vi "Start Stream.vi"(8 "error in (no error)":errorcluster, 10 "Camera Settings":T1={"Exposure Time (ms)"=100.0, "Binning"=enum."2x2", "Scan Mode"=0, "Frames to Acquire"=1000.0, "Pixel Correction"=FALSE, "Frames to Skip"=0, "File Path"=path "", "Duty cycle"=0.0, "ALEX"=FALSE, "Shutter Enable"=[], "fluidics trigger frame"=0, "Bit Depth"=16, "Image Width (px)"=0, "Image Height (px)"=0, "Horizontal Offset (px)"=0, "Vertical Offset (px)"=0} {"fluidics trigger frame" max=60000 step=1; "Exposure Time (ms)" min=1.0 max=10000.0 step=1.0}, 11 "Camera in":refnum<class "Camera.lvclass">) -> (0 "error out":errorcluster, 3 "Camera out":refnum<class "Camera.lvclass">)   [LabVIEW 2023, in "Camera.lvlib" / "Camera.lvclass"]
uses:
  Camera.lvclass
  Resources/Type Defs/Camera Settings.ctl
  Camera.lvclass/Camera.ctl
  <vilib>/Utility/error.llb/DialogType.ctl
  <vilib>/ActorFramework/Actor/Actor.lvclass/Actor.ctl
  <vilib>/ActorFramework/Message Enqueuer/Message Enqueuer.lvclass/Message Enqueuer.ctl
  <vilib>/ActorFramework/Message Enqueuer/Enqueue.vi
  Application Messages/Record Button Off Msg/Cancel Operation Msg.lvclass
  Resources/GLOBAL/GLOBAL Time-critical.vi
  <vilib>/ActorFramework/Message Priority Queue/Priority Enqueue.vi
  <vilib>/ActorFramework/Actor/Actor.lvclass
  <vilib>/ActorFramework/Message Enqueuer/Message Priority.ctl
  <vilib>/ActorFramework/Message Enqueuer/Message Enqueuer.lvclass
  Camera Messages/Get Most Recent Frame (if active) Msg/Get Most Recent Frame (if active) Msg.lvclass
  C:/FlashGordon/Development/Hardware/Device/Device.lvclass
  C:/Program Files/National Instruments/LabVIEW 2023/vi.lib/ActorFramework/Actor/Actor.lvclass
  C:/FlashGordon/Development/Hardware/Camera/Camera.lvclass
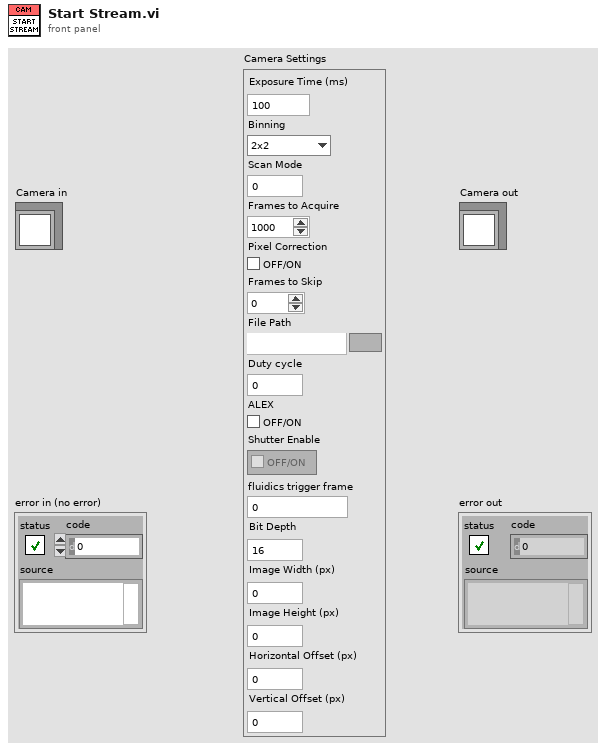
[diagram p1: front panel]
types:
  T1 = typedef "Camera Settings.ctl" = cluster{"Exposure Time (ms)":dbl, "Binning":enum16{"1x1", "2x2", "4x4"}, "Scan Mode":i32, "Frames to Acquire":dbl, "Pixel Correction":bool, "Frames to Skip":u32, "File Path":path, "Duty cycle":dbl, "ALEX":bool, "Shutter Enable":bool[], "fluidics trigger frame":u16, "Bit Depth":u16, "Image Width (px)":u16, "Image Height (px)":u16, "Horizontal Offset (px)":u16, "Vertical Offset (px)":u16}
  T2 = typedef "Actor Framework.lvlib/Message Enqueuer.lvclass/Message Priority.ctl" = enum16{"Low", "Normal", "High"}
  T3 = enum16{"open", "replace", "create", "open or create", "replace or create", "replace or create with confirmation"}
  T4 = typedef "DialogType.ctl" = u16
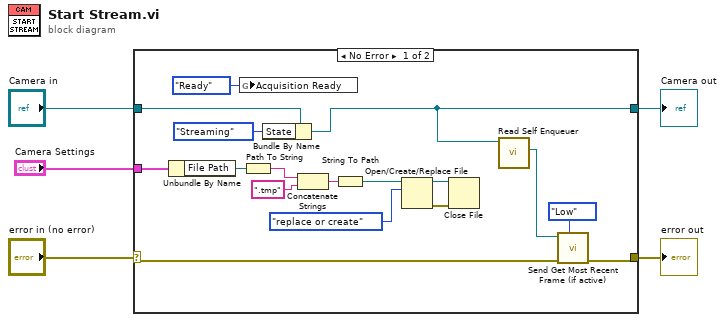
[diagram p0: block diagram]
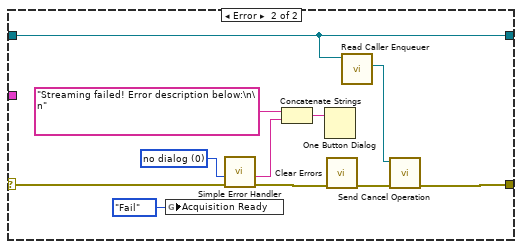
[diagram p2: hidden frame]
diagram:
  n1 = case shown="No Error" "error in (no error)" {
    selector: "error in (no error)" -> [w7 w26]
    tunnel: [w6 w25] -> w4
    tunnel: [w9 w24] -> w2
    tunnel: "Camera in" -> [w12 w24]
    tunnel: "Camera Settings" -> [w21 _]
    frame No Error {
      n2 = Unbundle By Name(w21) -> ("File Path"=w14:path)
      n3 = global write "GLOBAL Time-critical.vi" "Acquisition Ready"(enum16{"Waiting", "Ready", "Fail", "Timeout"}."Ready" ("Acquisition Ready")) -> ()
      n4 = Path To String(path=w14) -> (string=w17:string)
      n5 = Bundle By Name(cluster=w12, "State"=enum16{"Idle", "Live Mode", "Streaming"}."Streaming") -> (w9:refnum<class "Camera.lvclass">)
      n6 = Concatenate Strings(w17, ".tmp" ("string")) -> (w15:string)
      n7 = String To Path(string=w15) -> (path=w13:path)
      n8 = Open/Create/Replace File(file path (use dialog)=w13, operation (0:open)=T3."replace or create") -> (refnum out=w20:refnum<file>, error out=w19:errorcluster)  [unwired: 4 in, 1 out]
      n9 = Close File(refnum=w20, error in=w19) -> ()  [unwired: 2 out]
      n10 = call <vilib>:"Read Self Enqueuer.vi"("Actor"=w9) -> ("Self Enqueuer"=w8:refnum<class "Message Enqueuer.lvclass">)  [unwired: 10 in]
      n11 = call "Send Get Most Recent Frame (if active).vi"("Message Priority (Normal)"=Message_Priority."Low", "error in (no error)"=w7, "Message Enqueuer"=w8) -> ("error out"=w6:errorcluster)  [unwired: 7 in, 1 out]
    }
    frame Error {
      w32 = T4 0 items=["no dialog", "OK message", "continue or stop message", "OK message + warnings", "continue/stop + warnings"] ("type of dialog (OK msg:1)")
      n12 = global write "GLOBAL Time-critical.vi" "Acquisition Ready"(enum16{"Waiting", "Ready", "Fail", "Timeout"}."Fail" ("Acquisition Ready")) -> ()
      n13 = call <vilib>:"Simple Error Handler.vi"("type of dialog (OK msg:1)"=w32, "error in (no error)"=w26) -> ("source out"=w30:string, "error out"=w33:errorcluster)  [unwired: 3 in, 3 out]
      n14 = Concatenate Strings("Streaming failed! Error description below:\n\n" ("string"), w30) -> (w31:string)
      n15 = One Button Dialog(message=w31) -> ()  [unwired: 1 in, 1 out]
      n16 = call <vilib>:"Clear Errors.vi"("error in (no error)"=w33) -> ("error out"=w28:errorcluster)  [unwired: 5 in, 1 out]
      n17 = call <vilib>:"Read Caller Enqueuer.vi"("Actor"=w24) -> ("Caller Enqueuer"=w27:refnum<class "Message Enqueuer.lvclass">)  [unwired: 10 in]
      n18 = call "Send Cancel Operation.vi"("error in (no error)"=w28, "Message Enqueuer"=w27) -> ("error out"=w25:errorcluster)  [unwired: 8 in, 1 out]
    }
  }
  "error out" <- w4
  "Camera out" <- w2
